vi "ecg_ncs_v1e.vi"() -> ()   [LabVIEW 2016]
uses:
  <instrlib>/niUSRP/niUSRP Timestamp.ctl
  C:/Program Files/National Instruments/LabVIEW 2016/examples/Instrument IO/Serial/support/Serial - Settings.ctl
  <vilib>/Analysis/coordinate.llb/Wrap Angle (array).vi
  <instrlib>/niUSRP/niUSRP Configure Time Start Trigger.vi
  <vilib>/Analysis/3filter.llb/Butterworth Filter (DBL).vi
  <vilib>/Instr/_visa.llb/VISA Configure Serial Port (Instr).vi
  <instrlib>/niUSRP/niUSRP Write Tx Data (2D CDB).vi
  <instrlib>/niUSRP/niUSRP Fetch Rx Data (2D CDB).vi
  <vilib>/measure/NI_MABase.lvlib
  <vilib>/Analysis/NI_AALBase.lvlib
  <vilib>/Analysis/NI_AALPro.lvlib
  <vilib>/Analysis/NI_AAL_Angle.lvlib
panel:
  out "size(s) 5":i32=800
  in  "Stop":bool
  out "size(s) 4":i32=800
  out "x/y":dbl=2000.0
  out "size(s) 3":i32=20000
  out "size(s) 2":i32=10
  out "Poor Sensor Quality: \nSensor off":bool=TRUE
  out "Poor Sensor Quality: \nSensor on":bool
  out "Heart Rate 2":u16[](array[numeric])=[71]
  out "Stop Loop":bool
  out "Loop index":i32=135
  out "size(s)":i32=384
  in  "Read Count":u32=800
  out "return count":u32=800
  out "Serial Settings:Number of Bytes at Serial Port":u32=8
  in  "Serial Settings":T1={"baud rate"=57600, "data bits"=8, "parity"=enum."None", "stop bits"=10, "flow control"=0} {"flow control" items=["None"=0, "XON/XOFF"=1, "RTS/CTS"=2, "DTR/DSR"=4]; "stop bits" items=["1.0"=10, "1.5"=15, "2.0"=20]; "data bits" min=5 max=8 step=1; "baud rate" items=["75"=75, "110"=110, "134"=134, "150"=150, "300"=300, "600"=600, "1200"=1200, "1800"=1800, "2400"=2400, "4800"=4800, "7200"=7200, "9600"=9600, "14400"=14400, "19200"=19200, "28800"=28800, "38400"=38400, "56000"=56000, "57600"=57600, "115200"=115200, "128000"=128000, "230400"=230400]}
  in  "VISA resource name":refnum<visa-resource-name>="bmd101"
  in  "?":enum32{"ECG", "Heart Rate"}(tab)
  out "?":i16(graph)=77
  out "?":u8[](graph)=[71]
  in  "File Name":string="Test"
  in  "order1":i32=5
  in  "Path":path=path "D:/Research/SummerFall17Spring18/CnC/NCS/EcgNcsCorrelation"
  in  "Low-Pass Freq":dbl=200.0 format="%#_13g"
  in  "Sampling Rate":i32=500
  out "Gain":dbl=-15.0
  out "Bandwidth":dbl=56000000.0
  out "Coerced Carrier Frequency":dbl=2000000000.0 format="%#.17g"
  out "Coerced Tx IQ rate":dbl=1000000.0
  out "Coerced Rx IQ rate":dbl=1000000.0
  out "error IO":errorcluster={"status"=FALSE, "code"=-1074118647, "source"=""}
  in  "Rx Number of Samples":i32=20000
  in  "Tab Control 2":enum32{"NI-294x/295x", "NI-2900/2901"}(tab)=enum."NI-2900/2901"
  in  "channel 0 carrier\n frequency [Hz]":dbl=2000000000.0 format="%#_6p"
  in  "Rx carrier frequency [Hz]":dbl=2000000000.0 format="%#_6p"
  in  "Tx carrier frequency [Hz]":dbl=1000000000.0 format="%#_6p"
  in  "Start Trigger Time":T2={"whole seconds"=1, "fractional seconds"=0.0}
  out "Tx Active Antenna":string="TX1"
  in  "Tab Control":T3(tab)
  out "NCS tag Amp":dbl[](graph)=[0.011680657018198379]
  out "NCS tag Phase":dbl[](graph)=[-1.312166394909216]
  out "Tag Amp":dbl[](graph)
  out "Tag Phase":dbl[](graph)
  out "Tx Waveform Graph":waveform(dbl)[](graph)
  in  "Channel 0\nTone Amplitude":dbl=0.707 step=0.05 format="%#.6g"
  in  "Channel 0 \nTone Frequency":dbl=5000.0 format="%#_6p"
  in  "Waveform Size":dbl=20000.0
  in  "Rx Active Antenna":string="RX2"
  in  "Device Name":refnum<k15>="MyB200"
  in  "Tx Gain":dbl=28.0 format="%#_6f"
  in  "Tx IQ Rate":dbl=1000000.0 format="%#_6p"
  in  "Rx Gain":dbl=32.0 format="%#_6f"
  in  "Rx IQ Rate":dbl=1000000.0 format="%#_6p"
  # "Rx Settings"
  # "Tx Settings"
  # "Note that on the NI-2900 and NI-2901, both Rx channels share an LO and both Tx channels share an LO. However, on the NI-294x/295x devices, Rx and Tx of channel 0 share an LO and Rx and Tx of channel 1 share an LO."
  # "This Tx graph should always have end and start tied up since this is being sent in a loop continuously. Otherwise phase jumps will be noticed."
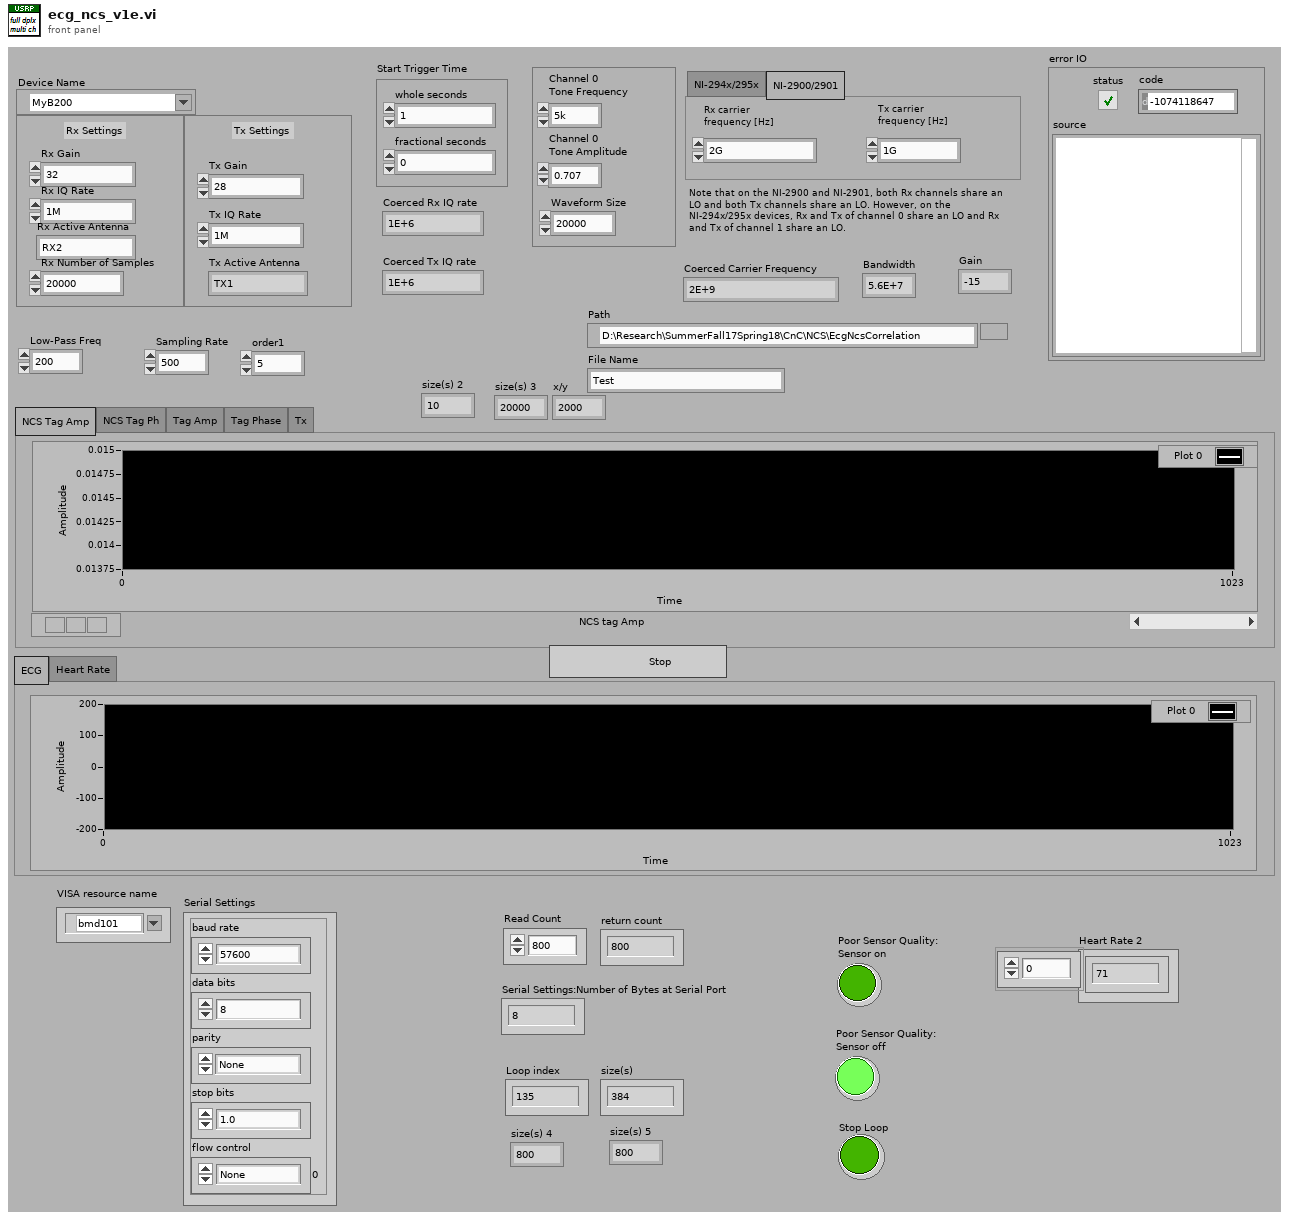
[diagram p1: front panel]
types:
  T1 = typedef "Serial - Settings.ctl" = cluster{"baud rate":u32, "data bits":u16, "parity":enum16{"None", "Odd", "Even", "Mark", "Space"}, "stop bits":u16, "flow control":u16}
  T2 = typedef "niUSRP Timestamp.ctl" = cluster{"whole seconds":u64, "fractional seconds":dbl}
  T3 = enum32{"NCS Tag Amp", "NCS Tag Ph", "Tag Amp", "Tag Phase", "Tx"}
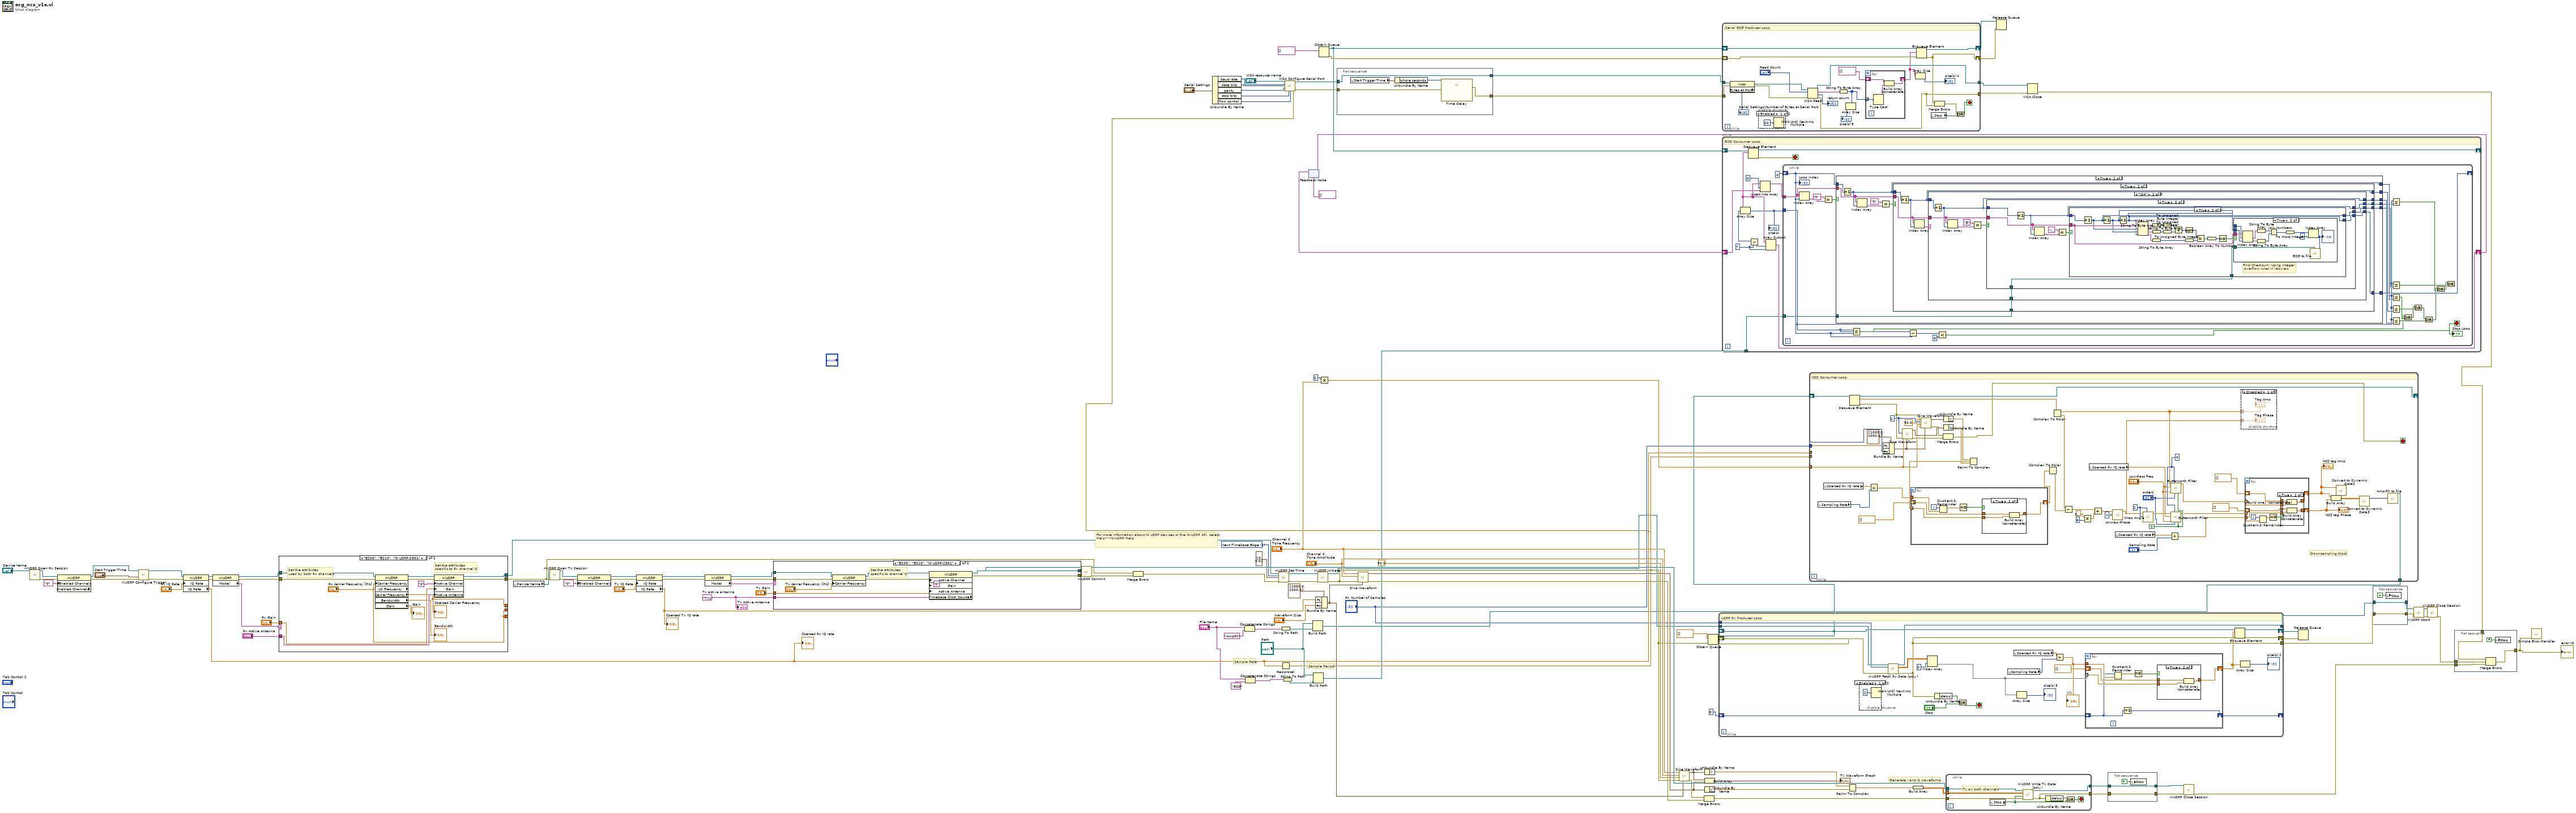
[diagram p0: block diagram]
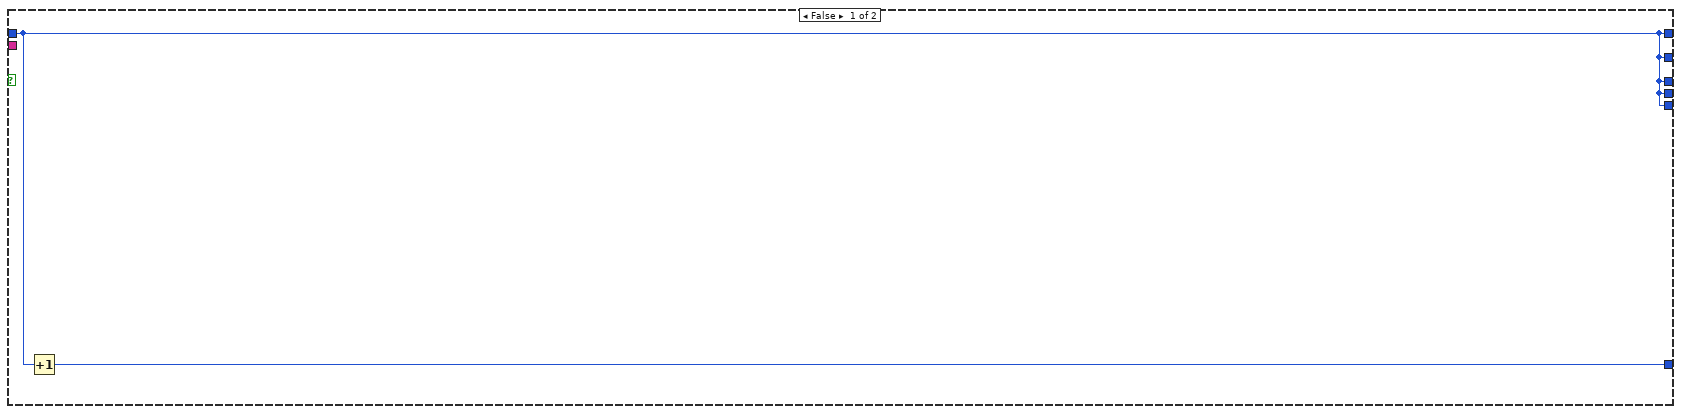
[diagram p4: hidden frame]
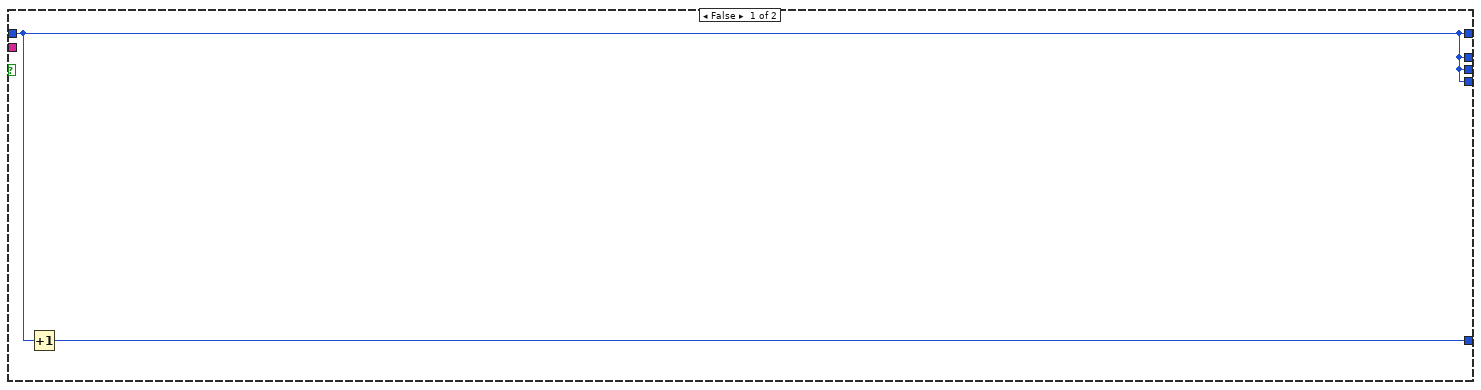
[diagram p5: hidden frame]
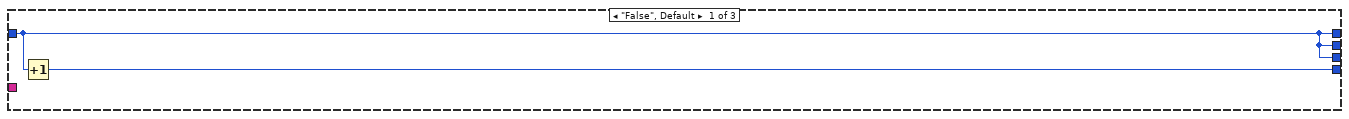
[diagram p6: hidden frame]
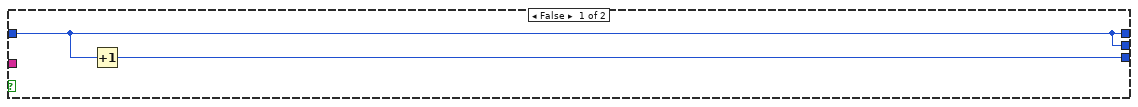
[diagram p7: hidden frame]
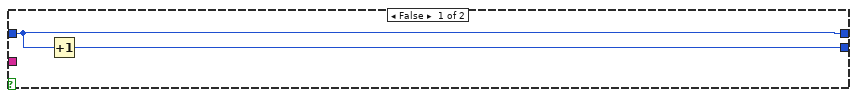
[diagram p8: hidden frame]
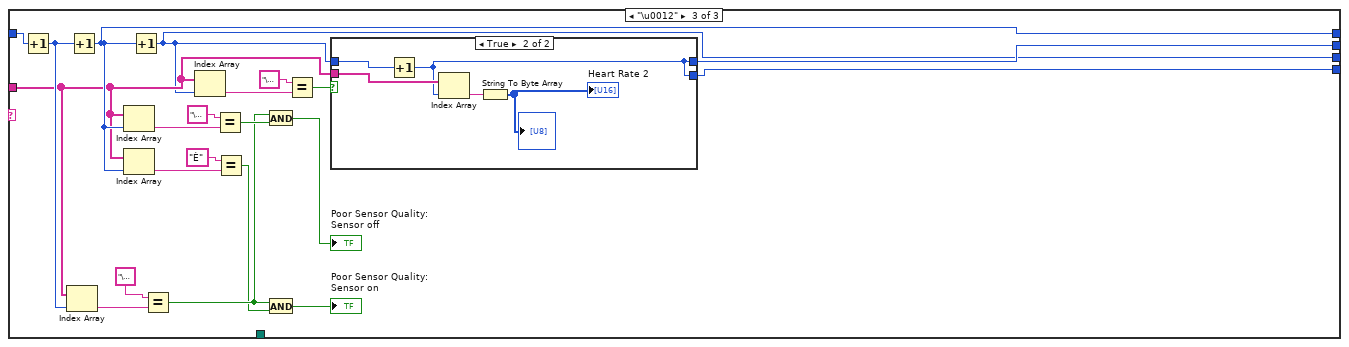
[diagram p10: hidden frame]
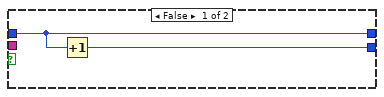
[diagram p11: hidden frame]
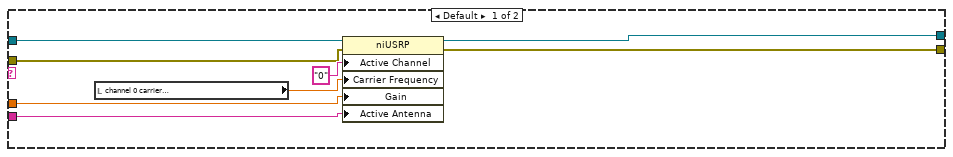
[diagram p13: hidden frame]
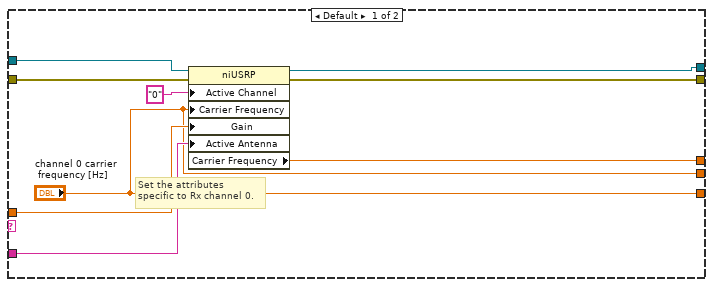
[diagram p14: hidden frame]
diagram:
  w91 = 1 items=["Now", "Next Timebase Edge"] ("apply timestamp")
  w60 = "TX1"  # Tx active antenna
  # "Sample Rate"
  # "Sample Period"
  # "For more information about NI USRP devices or the NI-USRP API, select Help>>NI-USRP Help."
  # "Generate I and Q waveforms."
  n1 = call <instrlib>:"niUSRP Open Rx Session.vi"("device names"="Device Name") -> ("session handle out"=w90:refnum<k15>, "error out"=w89:errorcluster)  [unwired: 13 in]
  n2 = property class="niUSRP" props=["Enabled Channels", "Enabled Channels"](reference=w90, error in=w89, "Enabled Channels"="0" ("Configuration:Enabled Channels")) -> (reference out=w88:refnum<k15>, error out=w87:errorcluster)  [unwired: 1 out]
  n3 = call-poly <instrlib>:"niUSRP Configure Trigger.vi"("session handle"=w88, "start trigger time"="Start Trigger Time", "error in (no error)"=w87) -> ("session handle out"=w84:refnum<k15>, "error out"=w83:errorcluster)  [unwired: 11 in]
  n4 = property class="niUSRP"(reference=w84, error in=w83, "IQ Rate"="Rx IQ Rate") -> (reference out=w80:refnum<k15>, error out=w81:errorcluster, "IQ Rate"=w20:dbl)
  "Coerced Rx IQ rate" <- w20
  n5 = property class="niUSRP"(reference=w80, error in=w81) -> (reference out=w75:refnum<k15>, error out=w76:errorcluster, "Model"=w77:string)
  n6 = case shown="\"B200\", \"B210\", \"NI USRP-2901\"" w77 {
    tunnel: w76 -> [w125 w135]
    tunnel: w75 -> [w124 w136]
    tunnel: [w121 w132] -> w79
    tunnel: [w120 w131] -> w78
    tunnel: "Rx Gain" -> [w123 w138]
    tunnel: "Rx Active Antenna" -> [w122 w137]
    tunnel: [w118 w127] -> _
    tunnel: ["channel 0 carrier\n frequency [Hz]" "Rx carrier frequency [Hz]"] -> _
    tunnel: ["channel 0 carrier\n frequency [Hz]" "Rx carrier frequency [Hz]"] -> _
    frame Default {
      # "Set the attributes \nspecific to Rx channel 0."
      n7 = property class="niUSRP"(reference=w124, error in=w125, "Active Channel"="0", "Carrier Frequency"="channel 0 carrier\n frequency [Hz]", "Gain"=w123, "Active Antenna"=w122) -> (reference out=w121:refnum<k15>, error out=w120:errorcluster, "Carrier Frequency"=w118:dbl)
    }
    frame "B200", "B210", "NI USRP-2901" {
      # "Set the attributes \nused by both Rx channels"
      # "Set the attributes \nspecific to Rx channel 0."
      n8 = property class="niUSRP" props=["Carrier Frequency", "LO Frequency", "Carrier Frequency", "Bandwidth", "Gain"](reference=w136, error in=w135, "Carrier Frequency"="Rx carrier frequency [Hz]") -> (reference out=w134:refnum<k15>, error out=w133:errorcluster, "Carrier Frequency"=w127:dbl, "Bandwidth"=→"Bandwidth":dbl, "Gain"=→"Gain":dbl)  [unwired: 1 out]
      "Coerced Carrier Frequency" <- w127
      n9 = property class="niUSRP"(reference=w134, error in=w133, "Active Channel"="0", "Gain"=w138, "Active Antenna"=w137) -> (reference out=w132:refnum<k15>, error out=w131:errorcluster)
    }
  }
  n10 = local read "Device Name"() -> (w112:refnum<k15>)
  n11 = call <instrlib>:"niUSRP Open Tx Session.vi"("device names"=w112, "error in (no error)"=w78) -> ("session handle out"=w86:refnum<k15>, "error out"=w85:errorcluster)  [unwired: 12 in]
  n12 = property class="niUSRP"(reference=w86, error in=w85, "Enabled Channels"="0" ("Configuration:Enabled Channels")) -> (reference out=w72:refnum<k15>, error out=w71:errorcluster)
  n13 = property class="niUSRP"(reference=w72, error in=w71, "IQ Rate"="Tx IQ Rate") -> (reference out=w66:refnum<k15>, error out=w67:errorcluster, "IQ Rate"=w64:dbl)
  "Coerced Tx IQ rate" <- w64
  n14 = property class="niUSRP"(reference=w66, error in=w67) -> (reference out=w68:refnum<k15>, error out=w69:errorcluster, "Model"=w65:string)
  n15 = case shown="\"B200\", \"B210\", \"NI USRP-2901\"" w65 {
    tunnel: "Tx Gain" -> [w147 w157]
    tunnel: w60 -> [w145 w155]
    tunnel: [w141 w149] -> w62
    tunnel: [w140 w148] -> w63
    tunnel: w69 -> [w144 w151]
    tunnel: w68 -> [w143 w154]
    frame Default {
      n16 = local read "channel 0 carrier\n frequency [Hz]"() -> (w142:dbl)
      n17 = property class="niUSRP"(reference=w143, error in=w144, "Active Channel"="0", "Carrier Frequency"=w142, "Gain"=w147, "Active Antenna"=w145) -> (reference out=w141:refnum<k15>, error out=w140:errorcluster)
    }
    frame "B200", "B210", "NI USRP-2901" {
      # "Set the attributes \nspecific to channel 0."
      n18 = property class="niUSRP"(reference=w154, error in=w151, "Carrier Frequency"="Tx carrier frequency [Hz]") -> (reference out=w153:refnum<k15>, error out=w152:errorcluster)
      n19 = property class="niUSRP" props=["Active Channel", "Gain", "Active Antenna", "Timebase Clock Source"](reference=w153, error in=w152, "Active Channel"="0", "Gain"=w157, "Active Antenna"=w155) -> (reference out=w149:refnum<k15>, error out=w148:errorcluster)  [unwired: 1 out]
    }
  }
  n20 = call <instrlib>:"niUSRP Commit.vi"("session handle"=w62, "error in (no error)"=w63) -> ("session handle out"=w114:refnum<k15>, "error out"=w115:errorcluster)  [unwired: 12 in]
  n21 = Merge Errors(w78, w115) -> (w93:errorcluster)
  n22 = Unbundle By Name("Serial Settings") -> ("baud rate"=w42:u32, "data bits"=w41:u16, "parity"=w40:enum16{"None", "Odd", "Even", "Mark", "Space"}, "stop bits"=w39:u16, "flow control"=w38:u16)
  n23 = Concatenate Strings("File Name", "AmpPh") -> (w46:string)
  n24 = Concatenate Strings("File Name", "ECG") -> (w23:string)
  n25 = call <instrlib>:"niUSRP Set Time.vi"("session handle"=w79, "apply timestamp"=w91, "timestamp"=T2 {"whole seconds"=0, "fractional seconds"=0.0}, "error in (no error)"=w93) -> ("session handle out"=w95:refnum<k15>, "error out"=w94:errorcluster)  [unwired: 10 in]
  n26 = String To Path(string=w46) -> (path=w45:path)
  n27 = Reciprocal(x=w20) -> (1/x=w98:dbl)
  n28 = String To Path(string=w23) -> (path=w22:path)
  n29 = feedback #1(string[] []) -> (w28:string[])
  n30 = Build Path(base path="Path", name or relative path=w45) -> (appended path=w2:path)
  n31 = Build Path(base path="Path", name or relative path=w22) -> (appended path=w25:path)
  n32 = Bundle By Name(cluster=cluster{"Fs":dbl, "#s":dbl} {"Fs"=1000.0, "#s"=1000.0} ("sampling info"), "Fs"=w64, "#s"="Waveform Size") -> (w97:cluster{"Fs":dbl, "#s":dbl})
  n33 = call <instrlib>:"niUSRP Initiate.vi"("session handle"=w95, "error in (no error)"=w94) -> ("session handle out"=w19:refnum<k15>, "error out"=w15:errorcluster)  [unwired: 12 in]
  n34 = call-poly "VISA Configure Serial Port"("VISA resource name"="VISA resource name", "baud rate (9600)"=w42, "data bits (8)"=w41, "parity (0:none)"=w40, "error in (no error)"=w15, "stop bits (10: 1 bit)"=w39, "flow control (0:none)"=w38) -> ("VISA resource name out"=w5:refnum<visa-resource-name>, "error out"=w7:errorcluster)  [unwired: 3 in, 4 out]
  n35 = Obtain Queue(element data type=string[] []) -> (queue out=w30:refnum<queue>, error out=w32:errorcluster)  [unwired: 4 in, 1 out]
  n36 = Multiply(x=2, y="Channel 0 \nTone Frequency") -> (x*y=w48:dbl)
  n37 = flat-sequence {
    tunnel: w7 -> [w160]
    tunnel: [w159] -> w6
    tunnel: w5 -> [w158]
    tunnel: [w158] -> w4
    frame #0 {
      n38 = local read "Start Trigger Time"() -> (w162:T2)
      n39 = Unbundle By Name(w162) -> ("whole seconds"=w161:u64)
      n40 = call "Time Delay"("error in (no error)"=w160, "Delay Time (s)"=w161) -> ("error out"=w159:errorcluster)  [unwired: 9 in]
    }
  }
  n41 = call <vilib>:"Sine Waveform.vi"("sampling info"=w97, "error in (no error)"=w15, "amplitude"="Channel 0\nTone Amplitude", "frequency"="Channel 0 \nTone Frequency") -> ("error out"=w59:errorcluster, "signal out"=w107:waveform(dbl))  [unwired: 6 in]
  n42 = call <vilib>:"Sine Waveform.vi"("sampling info"=w97, "error in (no error)"=w15, "phase"=90.0, "amplitude"="Channel 0\nTone Amplitude", "frequency"="Channel 0 \nTone Frequency") -> ("error out"=w58:errorcluster, "signal out"=w106:waveform(dbl))  [unwired: 5 in]
  n43 = Merge Errors(w58, w59) -> (w57:errorcluster)
  n44 = Unbundle By Name(w106) -> ("Y"=w105:dbl[])
  n45 = Build Array(w106, w107) -> (→"Tx Waveform Graph":waveform(dbl)[])
  n46 = Unbundle By Name(w107) -> ("Y"=w104:dbl[])
  n47 = Obtain Queue(element data type=dbl[] [], error in (no error)=w15) -> (queue out=w10:refnum<queue>, error out=w13:errorcluster)  [unwired: 3 in, 1 out]
  n48 = while {
    tunnel: w19 -> [w185]
    tunnel: [w184] -> w18
    tunnel: "Rx Number of Samples" -> [w183]
    tunnel: [w179] -> w9
    shift-right: [w181] -> w12
    shift-left: w10 -> [w182]
    shift-right: [w180] -> w11
    shift-left: w13 -> [w174]
    shift-right: [w163] -> _
    shift-left: 0 -> [w164]
    stop <- w170 stop-if-true
    # "USRP Rx Producer Loop"
    n49 = disable-structure shown="Enabled" {
      frame Enabled {
        n50 = Wait Until Next ms Multiple(millisecond multiple=u32 2 ("milliseconds to wait")) -> ()  [unwired: 1 out]
      }
      frame Disabled {
      }
    }
    n51 = call-poly <instrlib>:"niUSRP Fetch Rx Data (poly).vi"("session handle"=w185, "number of samples"=w183, "error in (no error)"=w174) -> ("session handle out"=w184:refnum<k15>, "data"=w177:cdb[][], "error out"=w179:errorcluster)  [unwired: 9 in, 1 out]
    n52 = Index Array(array=w177, index (row)=0 ("y")) -> (element=w165:cdb[])  [unwired: 1 in]
    n53 = Unbundle By Name(w179) -> ("status"=w171:bool)
    n54 = Or(x=w171, y="Stop") -> (x .or. y?=w170:bool)
    n55 = local read "Sampling Rate"() -> (w169:i32)
    n56 = local read "Coerced Rx IQ rate"() -> (w173:dbl)
    n57 = Array Size(array=w165) -> (size(s)=→"size(s) 3":i32)
    n58 = Divide(x=w173, y=w169) -> (x/y=w175:dbl)
    "x/y" <- w175
    n59 = for {
      tunnel: w165 -> [w193] mode=indexing
      shift-right: [w191] -> w168
      shift-left: dbl[] [] -> [w192]
      tunnel: w175 -> [w188]
      shift-right: [w186] -> w163
      shift-left: w164 -> [w187]
      n60 = Quotient & Remainder(x=w187, y=w188) -> (x-y*floor(x/y)=w189:dbl)  [unwired: 1 out]
      n61 = Increment(x=w187) -> (x+1=w186:i32)
      n62 = Equal To 0?(x=w189) -> (x = 0?=w190:bool)
      n63 = case shown="True" w190 {
        tunnel: w193 -> [_ w197]
        tunnel: w192 -> [w194 w196]
        tunnel: [w194 w195] -> w191
        frame False {
        }
        frame True {
          n64 = Build Array (concatenate)(w196, w197) -> (w195:cdb[])
        }
      }
    }
    n65 = Enqueue Element(queue=w182, element=w168, error in (no error)=w179) -> (queue out=w181:refnum<queue>, error out=w180:errorcluster)  [unwired: 1 in, 1 out]
    n66 = Array Size(array=w168) -> (size(s)=→"size(s) 2":i32)
  }
  n67 = while {
    shift-right: [w209] -> _
    shift-left: w30 -> [w210]
    shift-right: [w202] -> w29
    shift-left: w28 -> [w200]
    tunnel: w25 -> [w199]
    stop <- w208 stop-if-true
    w205 = 7
    # "ECG Consumer Loop"
    n68 = Dequeue Element(queue=w210) -> (queue out=w209:refnum<queue>, element=w203:string[], error out=w208:errorcluster)  [unwired: 2 in, 1 out]
    n69 = Array Size(array=w203) -> (size(s)=w207:i32)
    "size(s)" <- w207
    n70 = Subtract(x=w207, y=w205) -> (x-y=w206:i32)
    n71 = Insert Into Array(array=w203, index=0, new element=w200) -> (w204:string[])
    n72 = Array Subset(array=w203, index=w206, length=w205) -> (w202:string[])
    n73 = while {
      tunnel: w204 -> [w233]
      shift-right: [w237] -> _
      shift-left: 0 -> [w216]
      tunnel: w207 -> [w217]
      tunnel: w199 -> [w212]
      stop <- w213 stop-if-true
      n74 = Index Array(array=w233, index=w216) -> (element=w236:string)
      n75 = Equal?(x="ª", y=w236) -> (x = y?=w234:bool)
      n76 = case shown="True" w234 {
        tunnel: w216 -> [w238 w249]
        tunnel: [w239 w247] -> w237
        tunnel: w233 -> [_ w241]
        tunnel: [w238 w246] -> w232
        tunnel: [w238 w245] -> w230
        tunnel: [w238 w244] -> w227
        tunnel: [w238 w243] -> w224
        tunnel: [w238 w242] -> w221
        tunnel: w212 -> [_ w240]
        frame False {
          n77 = Increment(x=w238) -> (x+1=w239:i32)
        }
        frame True {
          n78 = Increment(x=w249) -> (x+1=w246:i32)
          n79 = Index Array(array=w241, index=w246) -> (element=w251:string)
          n80 = Equal?(x="ª", y=w251) -> (x = y?=w248:bool)
          n81 = case shown="True" w248 {
            tunnel: w246 -> [w252 w256]
            tunnel: [w253 w262] -> w247
            tunnel: w241 -> [_ w261]
            tunnel: [w252 w257] -> w245
            tunnel: [w252 w260] -> w244
            tunnel: [w252 w259] -> w243
            tunnel: [w252 w258] -> w242
            tunnel: w240 -> [_ w254]
            frame False {
              n82 = Increment(x=w252) -> (x+1=w253:i32)
            }
            frame True {
              n83 = Increment(x=w256) -> (x+1=w257:i32)
              n84 = Index Array(array=w261, index=w257) -> (element=w255:string)
              n85 = case shown="\"\\04\"" w255 {
                tunnel: w257 -> [w263 w271 w339]
                tunnel: [w264 w270 w321] -> w262
                tunnel: w261 -> [_ w269 w323]
                tunnel: [w263 w268 w325] -> w260
                tunnel: [w263 w267 w322] -> w259
                tunnel: [w263 w266 w320] -> w258
                tunnel: w254 -> [_ w265 _]
                frame "False", Default {
                  n86 = Increment(x=w263) -> (x+1=w264:i32)
                }
                frame "\u0004" {
                  n87 = Increment(x=w271) -> (x+1=w268:i32)
                  n88 = Index Array(array=w269, index=w268) -> (element=w272:string)
                  n89 = Equal?(x="€", y=w272) -> (x = y?=w273:bool)
                  n90 = case shown="True" w273 {
                    tunnel: w268 -> [w275 w282]
                    tunnel: [w276 w281] -> w270
                    tunnel: w269 -> [_ w280]
                    tunnel: [w275 w279] -> w267
                    tunnel: [w275 w278] -> w266
                    tunnel: w265 -> [_ w277]
                    frame False {
                      n91 = Increment(x=w275) -> (x+1=w276:i32)
                    }
                    frame True {
                      n92 = Increment(x=w282) -> (x+1=w279:i32)
                      n93 = Index Array(array=w280, index=w279) -> (element=w283:string)
                      n94 = Equal?(x="\u0002", y=w283) -> (x = y?=w284:bool)
                      n95 = case shown="True" w284 {
                        tunnel: w279 -> [w286 w292]
                        tunnel: [w287 w289] -> w281
                        tunnel: w280 -> [_ w293]
                        tunnel: [w286 w289] -> w278
                        tunnel: w277 -> [_ w288]
                        frame False {
                          n96 = Increment(x=w286) -> (x+1=w287:i32)
                        }
                        frame True {
                          # "Find Checksum: Using Integer\n overflow rules in labview"
                          n97 = Increment(x=w292) -> (x+1=w291:i32)
                          n98 = Increment(x=w291) -> (x+1=w290:i32)
                          n99 = Increment(x=w290) -> (x+1=w289:i32)
                          n100 = Index Array(array=w293, index #1=w291, index #2=w290, index #3=w289) -> (element #1=w307:string, element #2=w306:string, element #3=w300:string)
                          n101 = String To Byte Array(string=w307) -> (unsigned byte array=w305:u8[])
                          n102 = String To Byte Array(string=w306) -> (unsigned byte array=w304:u8[])
                          n103 = String To Byte Array(string=w300) -> (unsigned byte array=w299:u8[])
                          n104 = To Unsigned Byte Integer(number=w305) -> (unsigned 8bit integer=w303:u8[])
                          n105 = To Unsigned Byte Integer(number=w304) -> (unsigned 8bit integer=w302:u8[])
                          n106 = Add(x=w303, y=w302) -> (x+y=w301:u8[])
                          n107 = Not(x=w301) -> (.not. x?=w298:u8[])
                          n108 = To Unsigned Byte Integer(number=w299) -> (unsigned 8bit integer=w297:u8[])
                          n109 = Equal?(x=w298, y=w297) -> (x = y?=w296:bool[])
                          n110 = Boolean Array To Number(Boolean array=w296) -> (number=w295:u32)
                          n111 = Equal To 0?(x=w295) -> (x = 0?=w294:bool)
                          n112 = case shown="True" w294 {
                            tunnel: w293 -> [_ w319]
                            tunnel: w291 -> [_ w313]
                            tunnel: w290 -> [_ w312]
                            tunnel: w288 -> [_ w308]
                            frame False {
                            }
                            frame True {
                              n113 = Index Array(array=w319, index #1=w313, index #2=w312) -> (element #1=w318:string, element #2=w317:string)
                              n114 = String To Byte Array(string=w318) -> (unsigned byte array=w316:u8[])
                              n115 = String To Byte Array(string=w317) -> (unsigned byte array=w315:u8[])
                              n116 = Join Numbers(hi=w316, lo=w315) -> ((hi.lo)=w314:u16[])
                              n117 = To Word Integer(number=w314) -> (16bit integer=w311:i16[])
                              n118 = Index Array(array=w311, index=0) -> (element=w309:i16)
                              "?" <- w309
                              n119 = call "ECG to file"("Signals"=w309, "Filename"=w308) -> ()  [unwired: 15 in, 3 out]
                            }
                          }
                        }
                      }
                    }
                  }
                }
                frame "\u0012" {
                  n120 = Increment(x=w339) -> (x+1=w335:i32)
                  n121 = Index Array(array=w323, index=w335) -> (element=w338:string)
                  n122 = Increment(x=w335) -> (x+1=w325:i32)
                  n123 = Index Array(array=w323, index=w325) -> (element=w336:string)
                  n124 = Index Array(array=w323, index=w325) -> (element=w333:string)
                  n125 = Increment(x=w325) -> (x+1=w320:i32)
                  n126 = Equal?(x="\u0002", y=w338) -> (x = y?=w330:bool)
                  n127 = Index Array(array=w323, index=w320) -> (element=w326:string)
                  n128 = Equal?(x="\u0000", y=w336) -> (x = y?=w332:bool)
                  n129 = Equal?(x="È", y=w333) -> (x = y?=w329:bool)
                  n130 = And(x=w330, y=w332) -> (x .and. y?=→"Poor Sensor Quality: \nSensor off":bool)
                  n131 = And(x=w330, y=w329) -> (x .and. y?=→"Poor Sensor Quality: \nSensor on":bool)
                  n132 = Equal?(x="\u0003", y=w326) -> (x = y?=w324:bool)
                  n133 = case shown="True" w324 {
                    tunnel: w320 -> [w341 w347]
                    tunnel: w323 -> [_ w346]
                    tunnel: [w341 w345] -> w322
                    tunnel: [w342 w345] -> w321
                    frame False {
                      n134 = Increment(x=w341) -> (x+1=w342:i32)
                    }
                    frame True {
                      n135 = Increment(x=w347) -> (x+1=w345:i32)
                      n136 = Index Array(array=w346, index=w345) -> (element=w344:string)
                      n137 = String To Byte Array(string=w344) -> (unsigned byte array=→"Heart Rate 2" →"?":u8[])
                    }
                  }
                }
              }
            }
          }
        }
      }
      n138 = Less Or Equal?(x=w217, y=w216) -> (x <= y?=w218:bool)
      n139 = Subtract(x=w217, y=w216) -> (x-y=w215:i32)
      n140 = Less?(x=w215, y=6) -> (x < y?=w213:bool)
      "Stop Loop" <- w213
      n141 = Less Or Equal?(x=w217, y=w224) -> (x <= y?=w222:bool)
      n142 = Less Or Equal?(x=w217, y=w221) -> (x <= y?=w219:bool)
      n143 = Less Or Equal?(x=w217, y=w232) -> (x <= y?=w231:bool)
      n144 = Less Or Equal?(x=w217, y=w230) -> (x <= y?=w228:bool)
      n145 = Less Or Equal?(x=w217, y=w227) -> (x <= y?=w225:bool)
      n146 = Or(x=w218, y=w231) -> (x .or. y?=w229:bool)
      n147 = Or(x=w229, y=w228) -> (x .or. y?=w226:bool)
      n148 = Or(x=w226, y=w225) -> (x .or. y?=w223:bool)
      n149 = Or(x=w223, y=w222) -> (x .or. y?=w220:bool)
      n150 = Or(x=w220, y=w219) -> ()  [unwired: 1 out]
      "Loop index" <- w216
    }
  }
  n151 = feedback-in #1(w29) -> ()
  n152 = while {
    tunnel: w6 -> [w358]
    tunnel: [w362] -> w36
    shift-right: [w363] -> w34
    shift-left: w32 -> [w366]
    shift-right: [w364] -> w31
    shift-left: w30 -> [w365]
    tunnel: w4 -> [w360]
    tunnel: [w367] -> w35
    stop <- w369 stop-if-true
    # "Serial ECG Producer Loop"
    n153 = property class="Instr"(reference=w360, error in=w358) -> (reference out=w359:refnum<visa-resource-name>, error out=w357:errorcluster, "Bytes at Port"=→"Serial Settings:Number of Bytes at Serial Port":u32)
    n154 = disable-structure shown="Enabled" {
      frame Enabled {
        n155 = Wait Until Next ms Multiple(millisecond multiple=u32 20 ("milliseconds to wait")) -> ()  [unwired: 1 out]
      }
      frame Disabled {
      }
    }
    n156 = VISA Read(VISA resource name=w359, byte count="Read Count", error in (no error)=w357) -> (VISA resource name out=w367:refnum<visa-resource-name>, read buffer=w348:string, return count=→"return count":u32, error out=w362:errorcluster)
    n157 = String To Byte Array(string=w348) -> (unsigned byte array=w350:u8[])
    n158 = Array Size(array=w350) -> (size(s)=→"size(s) 5":i32)
    n159 = for {
      tunnel: w350 -> [w374] mode=indexing
      shift-right: [w372] -> w351
      shift-left: string[] [] -> [w373]
      n160 = Type Cast(x=w374) -> (*(type *) &x=w371:string)  [unwired: 1 in]
      n161 = Build Array (concatenate)(w373, w371) -> (w372:string[])
    }
    n162 = Array Size(array=w351) -> (size(s)=→"size(s) 4":i32)
    n163 = Enqueue Element(queue=w365, element=w351, error in (no error)=w366) -> (queue out=w364:refnum<queue>, error out=w363:errorcluster)  [unwired: 1 in, 1 out]
    n164 = local read "Stop"() -> (w355:bool)
    n165 = Merge Errors(w363, w362) -> (w361:errorcluster)
    n166 = Or(x=w361, y=w355) -> (x .or. y?=w369:bool)
  }
  n167 = while {
    tunnel: w98 -> [_]
    tunnel: "Rx Number of Samples" -> [w425]
    tunnel: w20 -> [w417]
    tunnel: w48 -> [w418]
    shift-right: [w386] -> _
    shift-left: w10 -> [w387]
    tunnel: w2 -> [w375]
    stop <- w381 stop-if-true
    w404 = 2 ("y")
    w398 = TRUE
    w400 = 0
    w423 = 1
    # "Downsampling block"
    # "NCS Consumer Loop"
    n168 = local read "Sampling Rate"() -> (w391:i32)
    n169 = local read "Coerced Rx IQ rate"() -> (w392:dbl)
    n170 = Dequeue Element(queue=w387) -> (queue out=w386:refnum<queue>, element=w385:dbl[], error out=w380:errorcluster)  [unwired: 2 in, 1 out]
    n171 = Divide(x=w392, y=w391) -> (x/y=w390:dbl)
    n172 = Bundle By Name(cluster=cluster{"Fs":dbl, "#s":dbl} {"Fs"=1000.0, "#s"=1000.0} ("sampling info"), "Fs"=w417, "#s"=w425) -> (w422:cluster{"Fs":dbl, "#s":dbl})
    n173 = call <vilib>:"Sine Waveform.vi"("sampling info"=w422, "error in (no error)"=w380, "amplitude"=w423, "frequency"=w418) -> ("error out"=w421:errorcluster, "signal out"=w426:waveform(dbl))  [unwired: 6 in]
    n174 = call <vilib>:"Sine Waveform.vi"("sampling info"=w422, "error in (no error)"=w380, "phase"=90.0, "amplitude"=w423, "frequency"=w418) -> ("error out"=w420:errorcluster, "signal out"=w419:waveform(dbl))  [unwired: 5 in]
    n175 = Merge Errors(w420, w421) -> (w381:errorcluster)
    n176 = Unbundle By Name(w419) -> ("Y"=w412:dbl[])
    n177 = Unbundle By Name(w426) -> ("Y"=w411:dbl[])
    n178 = Re/Im To Complex(1:w411, 2:w412) -> (0:w388:cdb[])
    n179 = for {
      tunnel: w388 -> [w434] mode=indexing
      shift-right: [w428] -> w384
      shift-left: dbl[] [] -> [w433]
      tunnel: w390 -> [w429]
      i -> [w432]
      n180 = Quotient & Remainder(x=w432, y=w429) -> (x-y*floor(x/y)=w430:dbl)  [unwired: 1 out]
      n181 = Equal To 0?(x=w430) -> (x = 0?=w431:bool)
      n182 = case shown="True" w431 {
        tunnel: w434 -> [_ w438]
        tunnel: w433 -> [w435 w437]
        tunnel: [w435 w436] -> w428
        frame False {
        }
        frame True {
          n183 = Build Array (concatenate)(w437, w438) -> (w436:cdb[])
        }
      }
    }
    n184 = Complex To Polar(r * e^(i*theta)=w384) -> (theta=w383:dbl[])  [unwired: 1 out]
    n185 = Complex To Polar(r * e^(i*theta)=w385) -> (r=w382:dbl[], theta=w402:dbl[])
    n186 = Subtract(x=w402, y=w383) -> (x-y=w406:dbl[])
    n187 = Multiply(x=3.141592653589793, y=6) -> (x*y=w407:dbl)
    n188 = local read "Coerced Rx IQ rate"() -> (w393:dbl)
    n189 = Add(x=w406, y=w407) -> (x+y=w405:dbl[])
    n190 = call <vilib>:"Unwrap Phase.vi"("phase unit"=1 ("y"), "Phase"=w405) -> ("Unwrapped Phase"=w403:dbl[])  [unwired: 8 in, 1 out]
    n191 = local read "Coerced Rx IQ rate"() -> (w415:dbl)
    n192 = call-poly <vilib>:"Wrap Angle.vi"("angle units"=w404, "angle range"=w404, "Angle In"=w403) -> ("Angle Out"=w401:dbl[])  [unwired: 7 in, 1 out]
    n193 = Divide(x=w415, y="Sampling Rate") -> (x/y=w413:dbl)
    n194 = call-poly <vilib>:"Butterworth Filter.vi"("init/cont (init:F)"=w398, "order"="order1", "filter type"=w400, "low cutoff freq: fl"="Low-Pass Freq", "sampling freq: fs"=w393, "X"=w382) -> ("Filtered X"=w394:dbl[])  [unwired: 2 in, 1 out]
    n195 = call-poly <vilib>:"Butterworth Filter.vi"("init/cont (init:F)"=w398, "order"="order1", "filter type"=w400, "low cutoff freq: fl"="Low-Pass Freq", "sampling freq: fs"=w393, "X"=w401) -> ("Filtered X"=w396:dbl[])  [unwired: 2 in, 1 out]
    n196 = disable-structure shown="Disabled" {
      disable-tunnel: w401 -> [w440 _]
      disable-tunnel: w382 -> [w439 _]
      frame Disabled {
        "Tag Amp" <- w439
        "Tag Phase" <- w440
      }
      frame Enabled {
      }
    }
    n197 = for {
      tunnel: w394 -> [w450] mode=indexing
      shift-right: [w448] -> w379
      shift-left: dbl[] [] -> [w449]
      tunnel: w413 -> [w444]
      shift-right: [w442] -> w378
      shift-left: dbl[] [] -> [w443]
      tunnel: w396 -> [w441] mode=indexing
      i -> [w447]
      n198 = Quotient & Remainder(x=w447, y=w444) -> (x-y*floor(x/y)=w445:dbl)  [unwired: 1 out]
      n199 = Equal To 0?(x=w445) -> (x = 0?=w446:bool)
      n200 = case shown="True" w446 {
        tunnel: w450 -> [_ w458]
        tunnel: w449 -> [w452 w457]
        tunnel: [w452 w456] -> w448
        tunnel: w443 -> [w451 w455]
        tunnel: [w451 w454] -> w442
        tunnel: w441 -> [_ w453]
        frame False {
        }
        frame True {
          n201 = Build Array (concatenate)(w457, w458) -> (w456:dbl[])
          n202 = Build Array (concatenate)(w455, w453) -> (w454:dbl[])
        }
      }
    }
    "NCS tag Amp" <- w379
    "NCS tag Phase" <- w378
    n203 = Build Array(w379, w378) -> (w376:dbl[][])
    n204 = call "Convert to Dynamic Data2"("Array"=w379) -> ()  [unwired: 3 in, 1 out]
    n205 = call "Convert to Dynamic Data3"("2D Array"=w376) -> ("Dynamic Data Type"=w377:dynamicdata)  [unwired: 3 in]
    n206 = call "Amp/Ph to file"("Signals"=w377, "Filename"=w375) -> ()  [unwired: 15 in, 3 out]
  }
  n207 = Re/Im To Complex(1:w104, 2:w105) -> (0:w100:cdb[])
  n208 = Build Array(w100) -> (w99:cdb[][])
  n209 = while {
    tunnel: w114 -> [w466]
    tunnel: w57 -> [w465]
    tunnel: [w463] -> w56
    tunnel: [w461] -> w53
    tunnel: w99 -> [w460]
    stop <- w462 stop-if-true
    # "Tx on both channels"
    n210 = local read "Stop"() -> (w459:bool)
    n211 = call-poly <instrlib>:"niUSRP Write Tx Data (poly).vi"("session handle"=w466, "data"=w460, "end of data?"=w459, "error in (no error)"=w465) -> ("session handle out"=w461:refnum<k15>, "error out"=w463:errorcluster)  [unwired: 10 in]
    n212 = Unbundle By Name(w463) -> ("status"=w464:bool)
    n213 = Compound Arithmetic op=OR(w464, w459) -> (w462:bool)
  }
  n214 = Release Queue(queue=w31, error in (no error)=w34) -> ()  [unwired: 1 in, 3 out]
  n215 = VISA Close(VISA resource name=w35, error in (no error)=w36) -> (error out=w26:errorcluster)
  n216 = flat-sequence {
    tunnel: [w468] -> w55
    tunnel: w56 -> [w468]
    tunnel: [w467] -> w54
    tunnel: w53 -> [w467]
    frame #0 {
      n217 = local write "Stop"(TRUE ("STOP")) -> ()
    }
  }
  n218 = call <instrlib>:"niUSRP Close Session.vi"("session handle"=w54, "error in (no error)"=w55) -> ("error out"=w52:errorcluster)  [unwired: 13 in]
  n219 = Release Queue(queue=w12, error in (no error)=w11) -> ()  [unwired: 1 in, 3 out]
  n220 = flat-sequence {
    tunnel: w18 -> [w471]
    tunnel: [w471] -> w17
    tunnel: w9 -> [w470]
    tunnel: [w470] -> w8
    frame #0 {
      n221 = local write "Stop"(TRUE ("STOP")) -> ()
    }
  }
  n222 = call <instrlib>:"niUSRP Abort.vi"("session handle"=w17, "error in (no error)"=w8) -> ("session handle out"=w111:refnum<k15>, "error out"=w110:errorcluster)  [unwired: 12 in]
  n223 = call <instrlib>:"niUSRP Close Session.vi"("session handle"=w111, "error in (no error)"=w110) -> ("error out"=w51:errorcluster)  [unwired: 13 in]
  n224 = flat-sequence {
    tunnel: w52 -> [w476]
    tunnel: [w475] -> w44
    tunnel: w51 -> [w474]
    tunnel: w26 -> [w473]
    frame #0 {
      n225 = Merge Errors(w473, w474, w476) -> (w475:errorcluster)
      n226 = local write "Stop"(FALSE ("STOP")) -> ()
    }
  }
  n227 = call <vilib>:"Simple Error Handler.vi"("error in (no error)"=w44) -> ()  [unwired: 1 in, 8 out]
  "Tx Active Antenna" <- w60
  "error IO" <- w44
